vi "Build.vi"(8 "error in (no error)":errorcluster, 10 "Pizza":refnum<class "Pizza(Product).lvclass">, 11 "SpicyPizzaBuilder in":refnum<class "SpicyPizzaBuilder.lvclass">) -> (0 "error out":errorcluster, 2 "Pizza out":refnum<class "Pizza(Product).lvclass">, 3 "SpicyPizzaBuilder out":refnum<class "SpicyPizzaBuilder.lvclass">)   [LabVIEW 2014, in "SpicyPizzaBuilder.lvclass"]
uses:
  SpicyPizzaBuilder.lvclass
  Pizza(Product)/Pizza(Product).lvclass
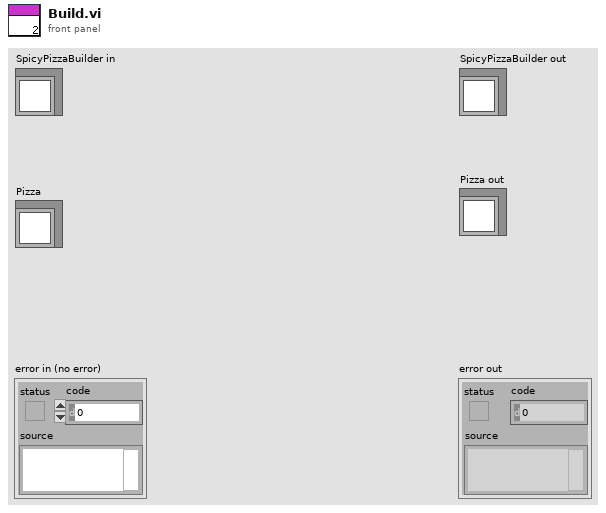
[diagram p1: front panel]
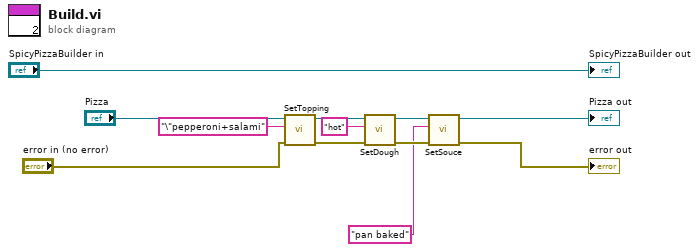
[diagram p0: block diagram]
diagram:
  n1 = call "SetTopping.vi"("error in (no error)"="error in (no error)", "Topping"="\"pepperoni+salami", "object in"="Pizza") -> ("error out"=w10:errorcluster, "object out"=w12:refnum<class "Pizza(Product).lvclass">)  [unwired: 7 in]
  n2 = call "SetDough.vi"("error in (no error)"=w10, "Dough"="hot", "object in"=w12) -> ("error out"=w9:errorcluster, "object out"=w11:refnum<class "Pizza(Product).lvclass">)  [unwired: 7 in]
  n3 = call "SetSouce.vi"("error in (no error)"=w9, "Souce"="pan baked", "object in"=w11) -> ("error out"=→"error out":errorcluster, "object out"=→"Pizza out":refnum<class "Pizza(Product).lvclass">)  [unwired: 7 in]
  "SpicyPizzaBuilder out" <- "SpicyPizzaBuilder in"
